vi "Get Property by Name.vi"(8 "error in":errorcluster, 10 "Property Name":string, 11 "VS CD API in":refnum<class "VS Custom Device API.lvclass">) -> (0 "error out":errorcluster, 2 "Value":variant, 3 "VS CDAPI out":refnum<class "VS Custom Device API.lvclass">)   [LabVIEW 2026, in "Template Engine.lvlib" / "VS Custom Device API.lvclass"]
uses:
  VS Custom Device API.lvclass
  VS Custom Device API.lvclass/VS Custom Device API.ctl
  <vilib>/NI VeriStand/Custom Device API/Custom Device API.lvlib
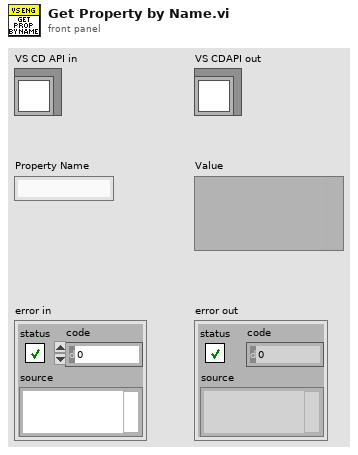
[diagram p1: front panel]
types:
  T1 = typedef "Custom Device API.lvlib/Custom Device Item Ref.ctl" = u64
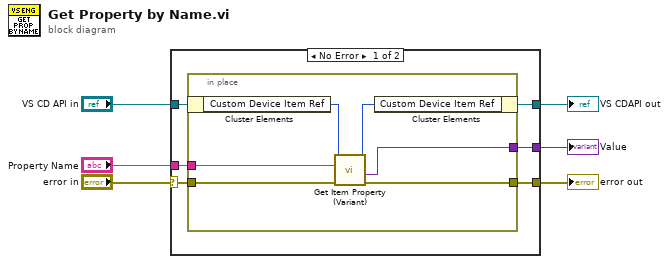
[diagram p0: block diagram]
diagram:
  n1 = case shown="No Error" "error in" {
    selector: "error in" -> [w12 w20]
    tunnel: "Property Name" -> [w11 _]
    tunnel: [w10 w20] -> w5
    tunnel: "VS CD API in" -> [w7 w19]
    tunnel: [w9 w19] -> w1
    tunnel: [w8 _] -> w4
    frame No Error {
      n2 = in-place {
        in-place-border: w12 -> [w18]
        in-place-border: w11 -> [w17]
        in-place-border: [w16] -> w10
        in-place-border: [w13] -> w8
        n3 = in-place-cluster #1(w7) -> ("Custom Device Item Ref"=w15:u64)
        n4 = call <vilib>:"Get Item Property (Variant).vi"("error in (no error)"=w18, "Property Name"=w17, "Item Ref in"=w15) -> ("error out"=w16:errorcluster, "Value"=w13:variant, "Item Ref out"=w14:T1)  [unwired: 5 in, 1 out]
        n5 = in-place-cluster #1("Custom Device Item Ref"=w14) -> (w9:refnum<class "VS Custom Device API.lvclass">)
      }
    }
    frame Error {
    }
  }
  "error out" <- w5
  "VS CDAPI out" <- w1
  "Value" <- w4
